vi "Get Analog Replay Settings.vi"(8 "error in (no error)":errorcluster, 11 "NodeID":u64) -> (0 "error out":errorcluster, 2 "Analog Replay Settings":T1 {"Voltage at max speed" min=0.0 max=10.0; "Max speed (RPM)" min=1.0; "Voltage at min speed" min=0.0 max=10.0; "Min speed (RPM)" min=0.0; "Voltage below min speed" min=0.0 max=10.0; "DAC bipolar range (V)" min=0.0001}, 3 "NodeID":u64)   [LabVIEW 2017, in "Engine Simulation Toolkit Scripting API.lvlib"]
uses:
  Engine Simulation Toolkit Scripting API.lvlib
  Analog Replay Settings.ctl
  Shared/Properties.vi
  <vilib>/NI Veristand/Custom Device API/Get Item Property (Double).vi
  <vilib>/NI Veristand/Custom Device API/Get Item Property (Boolean).vi
  Shared/Engine Simulation Toolkit Shared.lvlib
  <vilib>/NI Veristand/Custom Device API/Custom Device API.lvlib
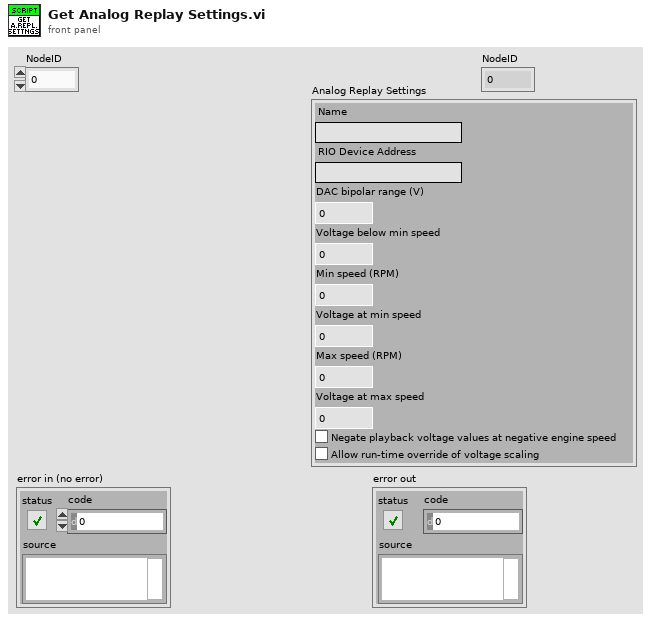
[diagram p1: front panel]
types:
  T1 = typedef "Engine Simulation Toolkit Scripting API.lvlib/Analog Replay Settings.ctl" = cluster{"Name":string, "RIO Device Address":string, "DAC bipolar range (V)":dbl, "Voltage below min speed":dbl, "Min speed (RPM)":dbl, "Voltage at min speed":dbl, "Max speed (RPM)":dbl, "Voltage at max speed":dbl, "ReverseNegate":bool, "VOverride":bool}
  T2 = typedef "Custom Device API.lvlib/Custom Device Item Info.ctl" = cluster{"Name":string, "Is Channel":bool, "GUID":string, "Is Waveform":bool}
  T3 = typedef "Custom Device API.lvlib/Custom Device Item Ref.ctl" = u64
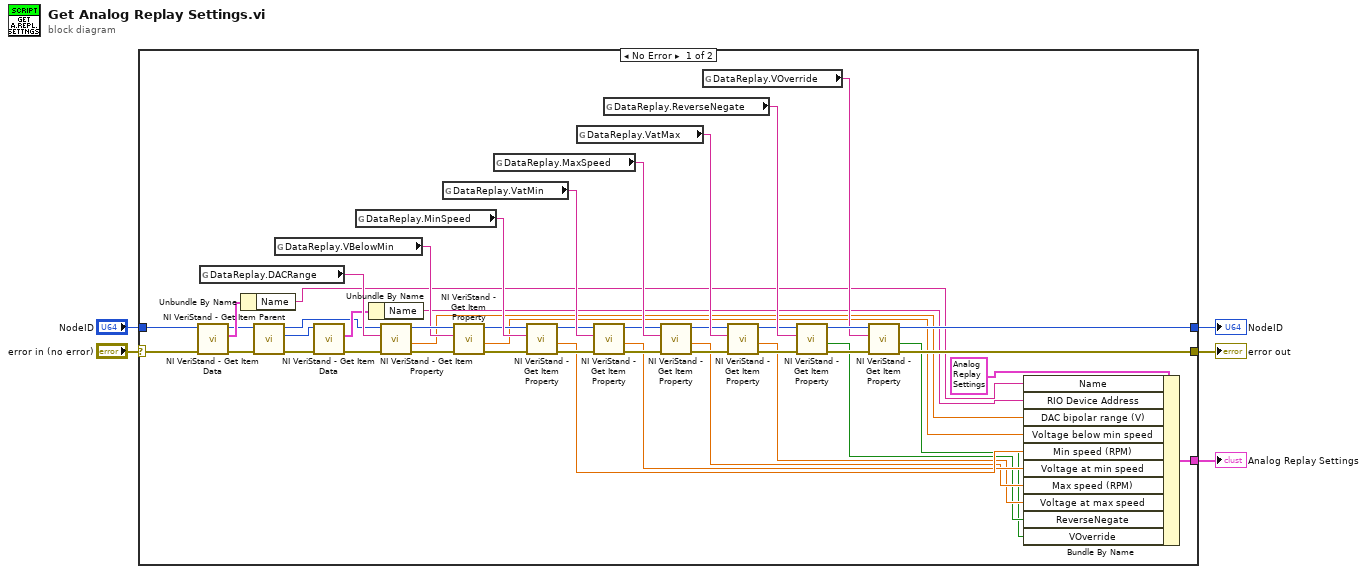
[diagram p0: block diagram]
diagram:
  n1 = case shown="No Error" "error in (no error)" {
    selector: "error in (no error)" -> [w10 w53]
    tunnel: [w51 w52] -> w5
    tunnel: [w49 w53] -> w4
    tunnel: [w26 _] -> w3
    tunnel: "NodeID" -> [w11 w52]
    frame No Error {
      n2 = call <vilib>:"NI VeriStand - Get Item Data.vi"("error in (no error)"=w10, "Item Ref in"=w11) -> ("error out"=w6:errorcluster, "Item Info"=w9:T2, "Item Ref out"=w7:T3)  [unwired: 6 in, 1 out]
      n3 = global read "Properties.vi" "DataReplay.DACRange"() -> (w28:string)
      n4 = Unbundle By Name(w9) -> ("Name"=w8:string)
      n5 = call <vilib>:"NI VeriStand - Get Item Parent.vi"("error in (no error)"=w6, "Item Ref in"=w7) -> ("error out"=w17:errorcluster, "Parent Ref"=w13:T3, "Item Ref out"=w12:T3)  [unwired: 6 in, 1 out]
      n6 = global read "Properties.vi" "DataReplay.VBelowMin"() -> (w29:string)
      n7 = call <vilib>:"NI VeriStand - Get Item Data.vi"("error in (no error)"=w17, "Item Ref in"=w13) -> ("error out"=w14:errorcluster, "Item Info"=w16:T2)  [unwired: 6 in, 2 out]
      n8 = global read "Properties.vi" "DataReplay.MinSpeed"() -> (w42:string)
      n9 = Unbundle By Name(w16) -> ("Name"=w15:string)
      n10 = call-poly <vilib>:"NI VeriStand - Get Item Property.vi"("error in (no error)"=w14, "Property Name"=w28, "Item Ref in"=w12) -> ("error out"=w31:errorcluster, "Value"=w25:dbl, "Item Ref out"=w30:T3)  [unwired: 5 in, 1 out]
      n11 = global read "Properties.vi" "DataReplay.VatMin"() -> (w43:string)
      n12 = call-poly <vilib>:"NI VeriStand - Get Item Property.vi"("error in (no error)"=w31, "Property Name"=w29, "Item Ref in"=w30) -> ("error out"=w32:errorcluster, "Value"=w24:dbl, "Item Ref out"=w37:T3)  [unwired: 5 in, 1 out]
      n13 = global read "Properties.vi" "DataReplay.MaxSpeed"() -> (w44:string)
      n14 = call-poly <vilib>:"NI VeriStand - Get Item Property.vi"("error in (no error)"=w32, "Property Name"=w42, "Item Ref in"=w37) -> ("error out"=w33:errorcluster, "Value"=w23:dbl, "Item Ref out"=w38:T3)  [unwired: 5 in, 1 out]
      n15 = global read "Properties.vi" "DataReplay.VatMax"() -> (w45:string)
      n16 = call-poly <vilib>:"NI VeriStand - Get Item Property.vi"("error in (no error)"=w33, "Property Name"=w43, "Item Ref in"=w38) -> ("error out"=w34:errorcluster, "Value"=w22:dbl, "Item Ref out"=w39:T3)  [unwired: 5 in, 1 out]
      n17 = global read "Properties.vi" "DataReplay.ReverseNegate"() -> (w46:string)
      n18 = call-poly <vilib>:"NI VeriStand - Get Item Property.vi"("error in (no error)"=w34, "Property Name"=w44, "Item Ref in"=w39) -> ("error out"=w35:errorcluster, "Value"=w21:dbl, "Item Ref out"=w40:T3)  [unwired: 5 in, 1 out]
      n19 = global read "Properties.vi" "DataReplay.VOverride"() -> (w47:string)
      n20 = call-poly <vilib>:"NI VeriStand - Get Item Property.vi"("error in (no error)"=w35, "Property Name"=w45, "Item Ref in"=w40) -> ("error out"=w36:errorcluster, "Value"=w20:dbl, "Item Ref out"=w41:T3)  [unwired: 5 in, 1 out]
      n21 = call-poly <vilib>:"NI VeriStand - Get Item Property.vi"("error in (no error)"=w36, "Property Name"=w46, "Item Ref in"=w41) -> ("error out"=w50:errorcluster, "Value"=w19:bool, "Item Ref out"=w48:T3)  [unwired: 5 in, 1 out]
      n22 = call-poly <vilib>:"NI VeriStand - Get Item Property.vi"("error in (no error)"=w50, "Property Name"=w47, "Item Ref in"=w48) -> ("error out"=w49:errorcluster, "Value"=w18:bool, "Item Ref out"=w51:T3)  [unwired: 5 in, 1 out]
      n23 = Bundle By Name(cluster=T1 {"Name"="", "RIO Device Address"="", "DAC bipolar range (V)"=0.0, "Voltage below min speed"=0.0, "Min speed (RPM)"=0.0, "Voltage at min speed"=0.0, "Max speed (RPM)"=0.0, "Voltage at max speed"=0.0, "ReverseNegate"=FALSE, "VOverride"=FALSE} ("Analog Replay Settings"), "Name"=w8, "RIO Device Address"=w15, "DAC bipolar range (V)"=w25, "Voltage below min speed"=w24, "Min speed (RPM)"=w23, "Voltage at min speed"=w22, "Max speed (RPM)"=w21, "Voltage at max speed"=w20, "ReverseNegate"=w19, "VOverride"=w18) -> (w26:T1)
    }
    frame Error {
    }
  }
  "error out" <- w4
  "Analog Replay Settings" <- w3
  "NodeID" <- w5
